vi "Unflatten.vi"(8 "error in (no error)":errorcluster, 11 "PC Reader in":refnum<class "PC Reader.lvclass">) -> (0 "error out":errorcluster, 3 "PC Reader out":refnum<class "PC Reader.lvclass">)   [LabVIEW 2015, in "PC Reader.lvclass"]
uses:
  PC Reader.lvclass
  PC Reader.lvclass/PC Reader.ctl
  Global/File Locations.vi
  Reader/Reader.lvclass
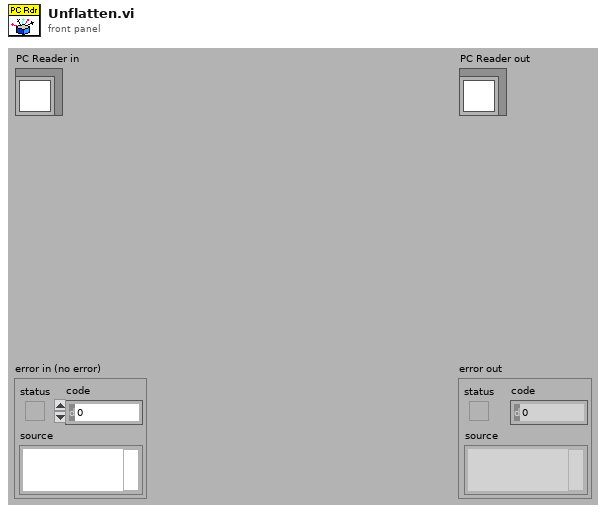
[diagram p1: front panel]
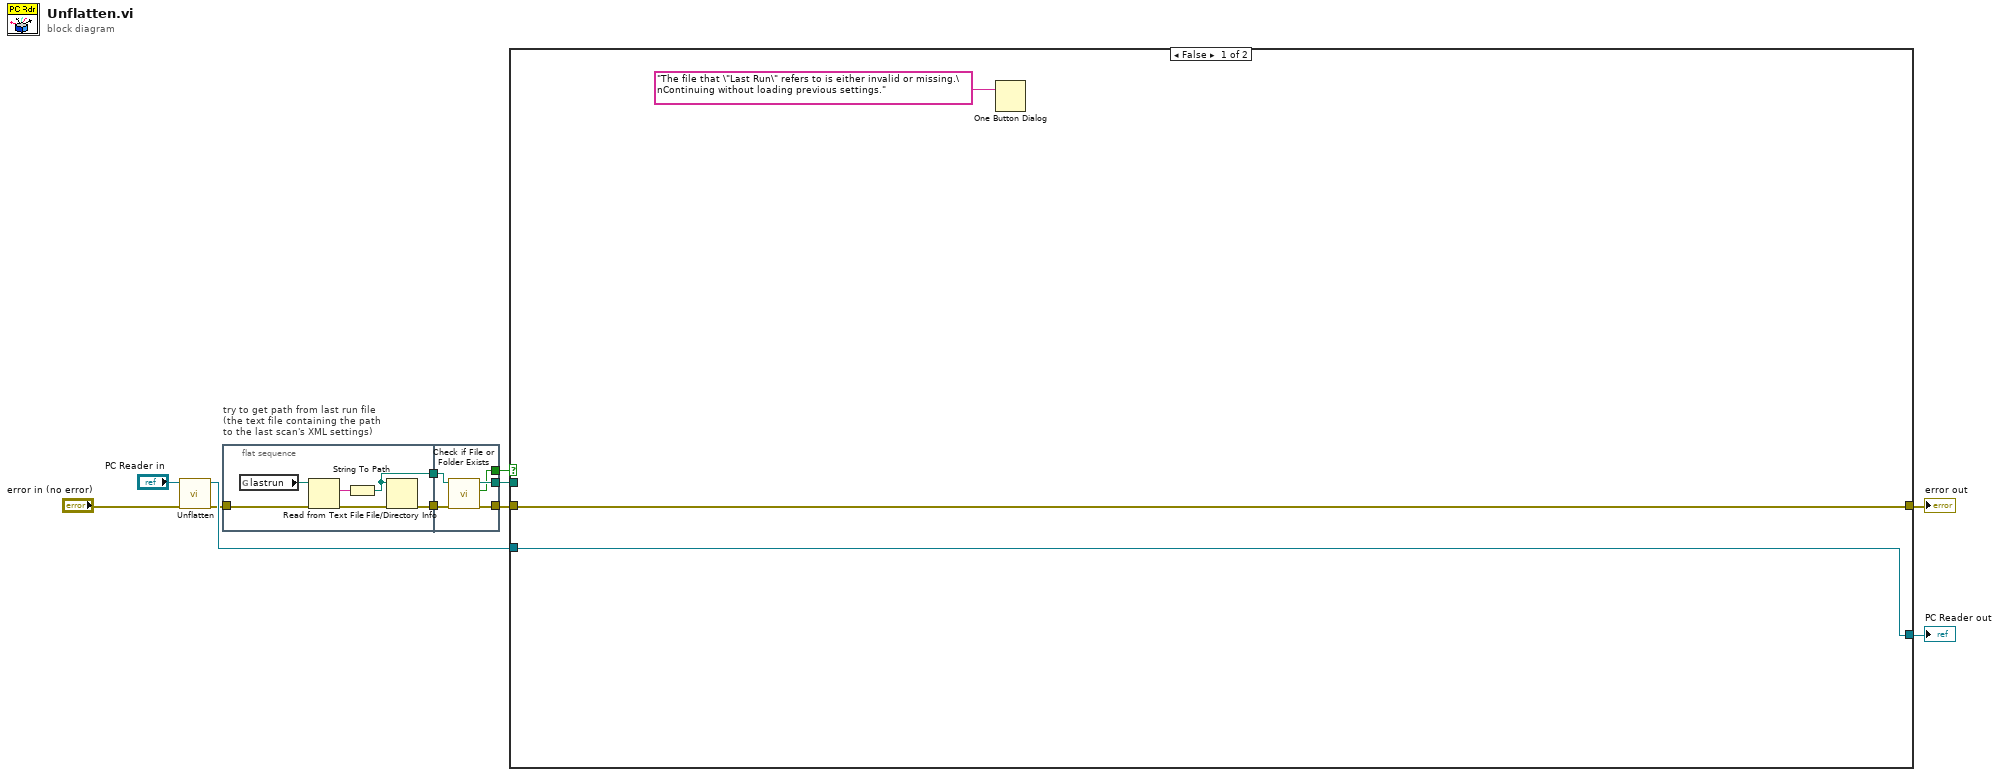
[diagram p0: block diagram]
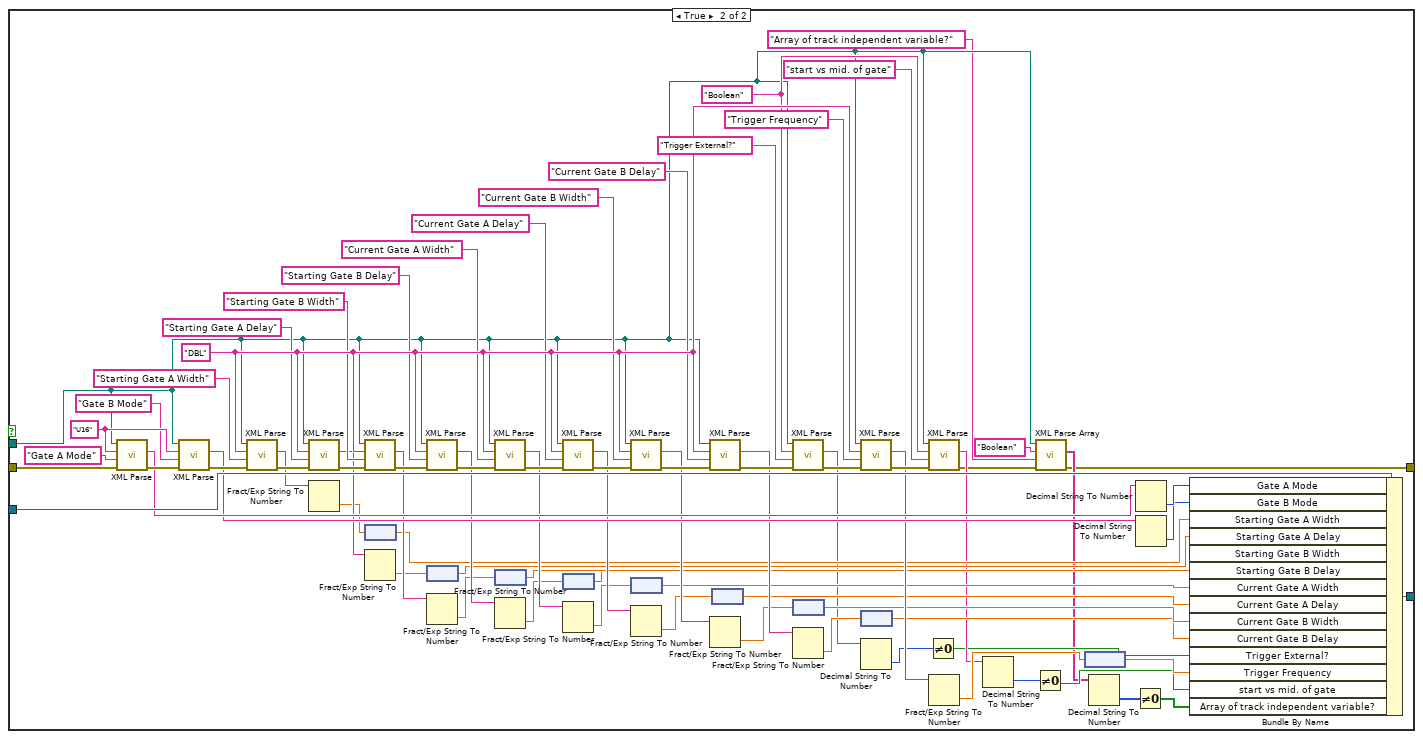
[diagram p2: hidden frame]
diagram:
  n1 = call-parent "Unflatten.vi"("error in (no error)"="error in (no error)", "Reader in"="PC Reader in") -> ("error out"=w7:errorcluster, "Reader out"=w11:refnum<class "PC Reader.lvclass">)  [unwired: 8 in]
  n2 = flat-sequence "try to get path from last run file\n(the text file containing the path\nto the last scan's XML settings)" {
    tunnel: w7 -> [w12]
    tunnel: [w17] -> w3
    tunnel: [w13] -> w2
    tunnel: [w21] -> w6
    tunnel: [w20] -> w5
    tunnel: w3 -> [w19]
    tunnel: w2 -> [w22]
    tunnel: [w18] -> w1
    frame #0 {
      n3 = global read "File Locations.vi" "lastrun"() -> (w15:path)
      n4 = Read from Text File(file (use dialog)=w15, error in=w12) -> (text=w16:string, error out=w14:errorcluster)  [unwired: 4 out]
      n5 = String To Path(string=w16) -> (path=w17:path)
      n6 = File/Directory Info(path=w17, error in=w14) -> (error out=w13:errorcluster)  [unwired: 6 out]
    }
    frame #1 {
      n7 = call <vilib>:"Check if File or Folder Exists.vi"("error in (no error)"=w22, "path"=w19) -> ("error out"=w21:errorcluster, "file or folder exists?"=w18:bool, "dup path"=w20:path)  [unwired: 7 in]
    }
  }
  n8 = case shown="False" w1 {
    tunnel: w11 -> [w23 w101]
    tunnel: [w23 w100] -> w8
    tunnel: w6 -> [w24 w99]
    tunnel: w5 -> [_ w33]
    tunnel: [w24 w26] -> w4
    frame False {
      n9 = One Button Dialog(message="The file that \"Last Run\" refers to is either invalid or missing.\nContinuing without loading previous settings.") -> ()  [unwired: 1 in, 1 out]
    }
    frame True {
      w74 = "Boolean"
      w83 = "DBL"
      w86 = "U16"
      n10 = call "XML Parse.vi"("error in (no error)"=w99, "Name String"="Gate A Mode", "Type String"=w86, "Path"=w33) -> ("error out"=w98:errorcluster, "String Out"=w70:string)  [unwired: 6 in]
      n11 = call "XML Parse.vi"("error in (no error)"=w98, "Name String"="Gate B Mode", "Type String"=w86, "Path"=w33) -> ("error out"=w97:errorcluster, "String Out"=w69:string)  [unwired: 6 in]
      n12 = call "XML Parse.vi"("error in (no error)"=w97, "Name String"="Starting Gate A Width", "Type String"=w83, "Path"=w33) -> ("error out"=w96:errorcluster, "String Out"=w66:string)  [unwired: 6 in]
      n13 = call "XML Parse.vi"("error in (no error)"=w96, "Name String"="Starting Gate A Delay", "Type String"=w83, "Path"=w33) -> ("error out"=w95:errorcluster, "String Out"=w65:string)  [unwired: 6 in]
      n14 = Fract/Exp String To Number(string=w66) -> (number=w57:dbl)  [unwired: 3 in, 1 out]
      n15 = call "XML Parse.vi"("error in (no error)"=w95, "Name String"="Starting Gate B Width", "Type String"=w83, "Path"=w33) -> ("error out"=w94:errorcluster, "String Out"=w64:string)  [unwired: 6 in]
      n16 = node(w57) -> (w56:dbl[unit])
      n17 = Fract/Exp String To Number(string=w65) -> (number=w55:dbl)  [unwired: 3 in, 1 out]
      n18 = call "XML Parse.vi"("error in (no error)"=w94, "Name String"="Starting Gate B Delay", "Type String"=w83, "Path"=w33) -> ("error out"=w93:errorcluster, "String Out"=w63:string)  [unwired: 6 in]
      n19 = node(w55) -> (w48:dbl[unit])
      n20 = Fract/Exp String To Number(string=w64) -> (number=w54:dbl)  [unwired: 3 in, 1 out]
      n21 = call "XML Parse.vi"("error in (no error)"=w93, "Name String"="Current Gate A Width", "Type String"=w83, "Path"=w33) -> ("error out"=w92:errorcluster, "String Out"=w62:string)  [unwired: 6 in]
      n22 = node(w54) -> (w47:dbl[unit])
      n23 = Fract/Exp String To Number(string=w63) -> (number=w53:dbl)  [unwired: 3 in, 1 out]
      n24 = call "XML Parse.vi"("error in (no error)"=w92, "Name String"="Current Gate A Delay", "Type String"=w83, "Path"=w33) -> ("error out"=w91:errorcluster, "String Out"=w61:string)  [unwired: 6 in]
      n25 = node(w53) -> (w46:dbl[unit])
      n26 = Fract/Exp String To Number(string=w62) -> (number=w52:dbl)  [unwired: 3 in, 1 out]
      n27 = call "XML Parse.vi"("error in (no error)"=w91, "Name String"="Current Gate B Width", "Type String"=w83, "Path"=w33) -> ("error out"=w90:errorcluster, "String Out"=w60:string)  [unwired: 6 in]
      n28 = node(w52) -> (w45:dbl[unit])
      n29 = Fract/Exp String To Number(string=w61) -> (number=w51:dbl)  [unwired: 3 in, 1 out]
      n30 = call "XML Parse.vi"("error in (no error)"=w90, "Name String"="Current Gate B Delay", "Type String"=w83, "Path"=w33) -> ("error out"=w89:errorcluster, "String Out"=w59:string)  [unwired: 6 in]
      n31 = Fract/Exp String To Number(string=w60) -> (number=w50:dbl)  [unwired: 3 in, 1 out]
      n32 = node(w51) -> (w44:dbl[unit])
      n33 = call "XML Parse.vi"("error in (no error)"=w89, "Name String"="Trigger External?", "Type String"=w74, "Path"=w33) -> ("error out"=w88:errorcluster, "String Out"=w38:string)  [unwired: 6 in]
      n34 = node(w50) -> (w43:dbl[unit])
      n35 = Fract/Exp String To Number(string=w59) -> (number=w49:dbl)  [unwired: 3 in, 1 out]
      n36 = call "XML Parse.vi"("error in (no error)"=w88, "Name String"="Trigger Frequency", "Type String"=w83, "Path"=w33) -> ("error out"=w87:errorcluster, "String Out"=w58:string)  [unwired: 6 in]
      n37 = node(w49) -> (w42:dbl[unit])
      n38 = Decimal String To Number(string=w38) -> (number=w37:i32)  [unwired: 2 in, 1 out]
      n39 = Not Equal To 0?(x=w37) -> (x != 0?=w34:bool)
      n40 = call "XML Parse.vi"("error in (no error)"=w87, "Name String"="start vs mid. of gate", "Type String"=w74, "Path"=w33) -> ("error out"=w32:errorcluster, "String Out"=w39:string)  [unwired: 6 in]
      n41 = Fract/Exp String To Number(string=w58) -> (number=w41:dbl)  [unwired: 3 in, 1 out]
      n42 = Decimal String To Number(string=w39) -> (number=w36:i32)  [unwired: 2 in, 1 out]
      n43 = Not Equal To 0?(x=w36) -> (x != 0?=w35:bool)
      n44 = call "XML Parse Array.vi"("error in (no error)"=w32, "Name String"="Array of track independent variable?", "Type String"="Boolean", "Path"=w33) -> ("error out"=w26:errorcluster, "Array"=w29:string[])  [unwired: 5 in]
      n45 = node(w41) -> (w40:dbl[unit])
      n46 = Decimal String To Number(string=w29) -> (number=w28:i32[])  [unwired: 2 in, 1 out]
      n47 = Not Equal To 0?(x=w28) -> (x != 0?=w27:bool[])
      n48 = Decimal String To Number(string=w70) -> (number=w68:i32)  [unwired: 2 in, 1 out]
      n49 = Decimal String To Number(string=w69) -> (number=w67:i32)  [unwired: 2 in, 1 out]
      n50 = Bundle By Name(cluster=w101, "Gate A Mode"=w68, "Gate B Mode"=w67, "Starting Gate A Width"=w56, "Starting Gate A Delay"=w48, "Starting Gate B Width"=w47, "Starting Gate B Delay"=w46, "Current Gate A Width"=w45, "Current Gate A Delay"=w44, "Current Gate B Width"=w43, "Current Gate B Delay"=w42, "Trigger External?"=w34, "Trigger Frequency"=w40, "start vs mid. of gate"=w35, "Array of track independent variable?"=w27) -> (w100:refnum<class "PC Reader.lvclass">)
    }
  }
  "PC Reader out" <- w8
  "error out" <- w4
